vi "DynamicRegistration.vi"() -> ()   [LabVIEW 2020]
panel:
  in  "stop":bool
  out "Web":string
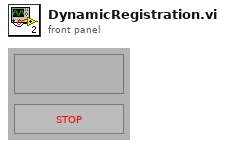
[diagram p1: front panel]
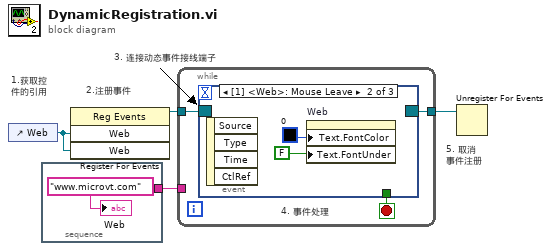
[diagram p0: block diagram]
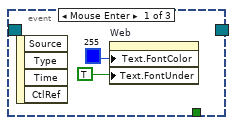
[diagram p2: hidden frame]
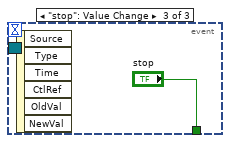
[diagram p3: hidden frame]
diagram:
  # "5. 取消\n事件注册"
  # "3. 连接动态事件接线端子"
  # "2.注册事件"
  # "1.获取控\n件的引用"
  n1 = control-ref of="Web"() -> (w1:refnum<vi>)
  n2 = stacked-sequence {
    tunnel: [w5] -> w2
    frame #0 {
      w5 = "www.microvt.com" ("String")
      "Web" <- w5
    }
  }
  n3 = register-events(w1, w1) -> (reference out=w4:refnum<event-registration>)  [unwired: 2 in, 1 out]
  n4 = while {
    tunnel: w4 -> [w8]
    tunnel: [w7] -> w3
    tunnel: w2 -> [_]
    stop <- w6 stop-if-true
    # "4. 事件处理"
    n5 = event shown="[1] <Web>: Mouse Leave" {
      selector: w8 -> [_ _ _]
      dyn-events: [_ _ _] -> w7
      timeout: _ -> [_ _ _]
      tunnel: [_ _ "stop"] -> w6
      event Mouse Enter {
        n6 = event-data() -> ()  [unwired: 5 out]
        n7 = property on="Web" class="Str"("Text.FontColor"=u32 255, "Text.FontUnder"=TRUE ("Text.Font:Underline")) -> ()  [unwired: 2 in, 2 out]
      }
      event Mouse Leave {
        n8 = event-data() -> ()  [unwired: 5 out]
        n9 = property on="Web" class="Str"("Text.FontColor"=u32 0, "Text.FontUnder"=FALSE ("Text.Font:Underline")) -> ()  [unwired: 2 in, 2 out]
      }
      event "stop": Value Change {
        n10 = event-data() -> ()  [unwired: 7 out]
      }
    }
  }
  n11 = Unregister For Events(event registration refnum=w3) -> ()  [unwired: 1 in, 1 out]
